vi "Destroy Test Executive.vi"(8 "error in (no error)":errorcluster, 11 "Test Executive in":refnum<class "Test Executive.lvclass">) -> (0 "error out":errorcluster)   [LabVIEW 2019, in "Test Executive.lvlib" / "Test Executive.lvclass"]
uses:
  <vilib>/gpm_packages/@cs/test-executive/Source/Test Executive/TestExecutive/Test Executive.lvclass
  <vilib>/gpm_packages/@cs/test-executive/Source/Test Executive/TestExecutive/Test Executive.lvclass/Test Executive.ctl
  <vilib>/gpm_packages/@cs/linked-list/Source/Linked List/Linked List Ref/Linked List Ref.lvclass
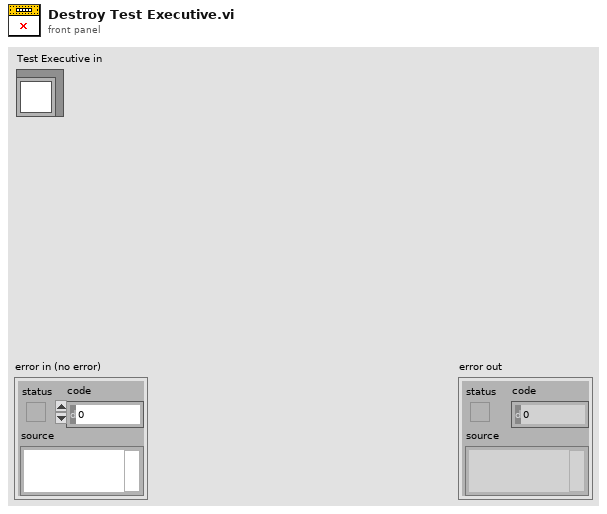
[diagram p1: front panel]
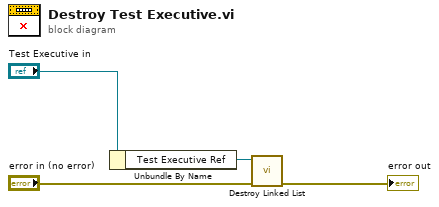
[diagram p0: block diagram]
diagram:
  n1 = Unbundle By Name("Test Executive in") -> ("Test Executive Ref"=w2:refnum<data-value>)
  n2 = call <vilib>:"Destroy Linked List.vi"("error in (no error)"="error in (no error)", "Linked List Ref"=w2) -> ("error out"=→"error out":errorcluster)  [unwired: 9 in]
